vi "Que Notifier send.vi"() -> ()   [LabVIEW 2022 SP3]
panel:
  in  "Nitification Send 2":bool
  in  "error in (no error)":errorcluster
  in  "stop":bool
  out "error out":errorcluster
  out "Sent Que":i32[](array[numeric])
  out "Sent Notifier":u8
  in  "Que Send":bool
  in  "Nitification Send":bool
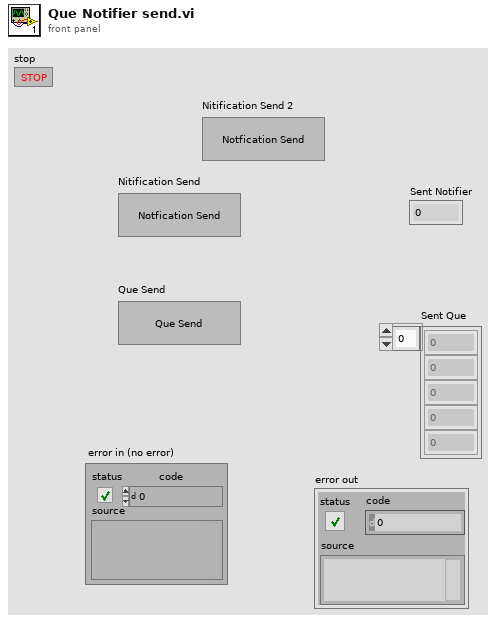
[diagram p1: front panel]
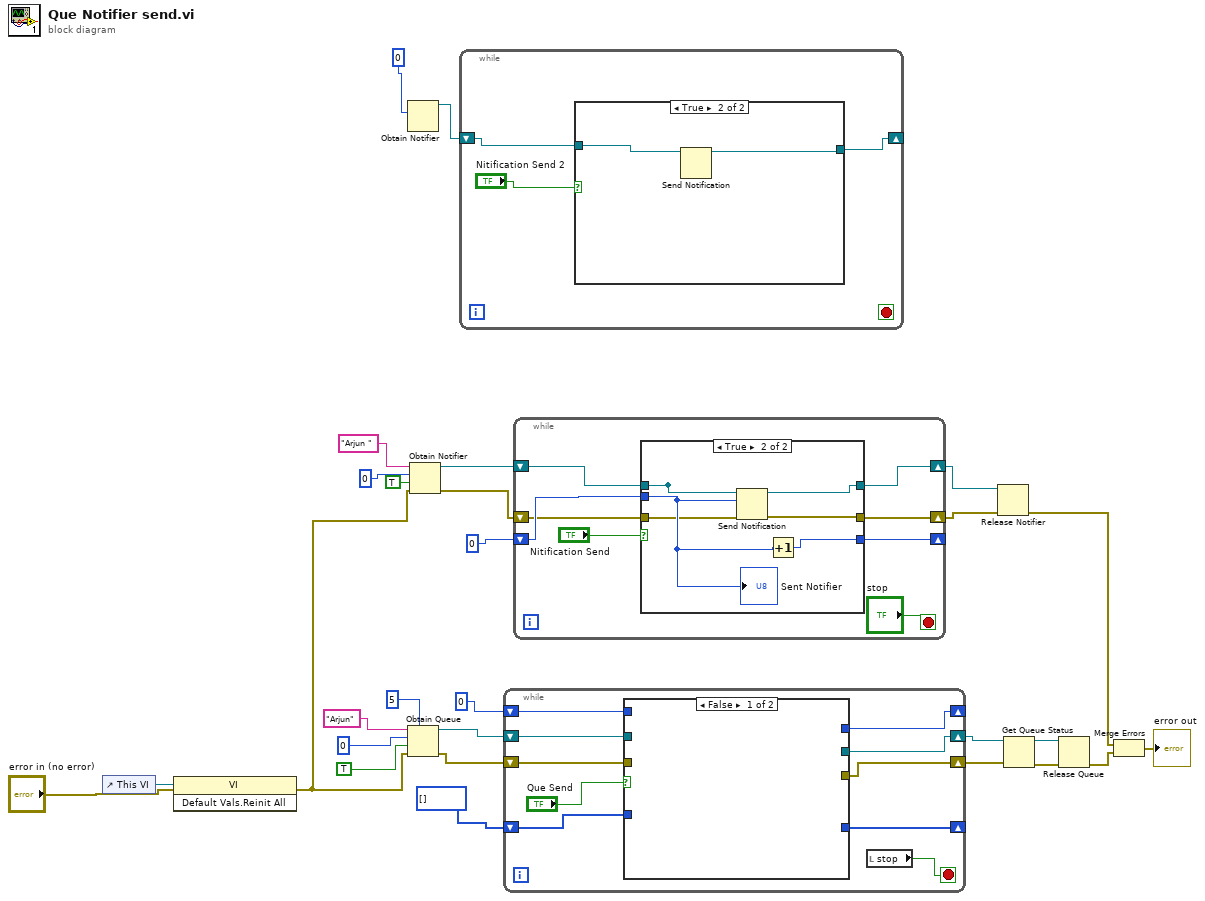
[diagram p0: block diagram]
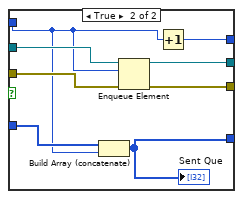
[diagram p3: hidden frame]
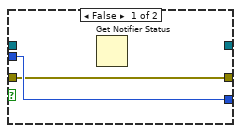
[diagram p4: hidden frame]
diagram:
  n1 = control-ref of="This VI"() -> (w10:refnum<vi>)
  n2 = invoke class="VI" method="Default Vals.Reinit All"(reference=w10, error in="error in (no error)") -> (error out=w9:errorcluster)  [unwired: 1 in, 2 out]
  n3 = Obtain Notifier(notification data type=0) -> (notifier out=w1:refnum<notifier>)  [unwired: 3 in, 2 out]
  n4 = Obtain Queue(max queue size (-1, unlimited)=5, name (unnamed)="Arjun", element data type=0, create if not found? (T)=TRUE, error in (no error)=w9) -> (queue out=w25:refnum<queue>, error out=w24:errorcluster)  [unwired: 1 out]
  n5 = Obtain Notifier(name (unnamed)="Arjun ", notification data type=0, create if not found? (T)=TRUE, error in (no error)=w9) -> (notifier out=w3:refnum<notifier>, error out=w8:errorcluster)  [unwired: 1 out]
  n6 = while {
    shift-right: [w29] -> _
    shift-left: w1 -> [w30]
    stop <- _ stop-if-true
    n7 = case shown="True" "Nitification Send 2" {
      tunnel: w30 -> [w32 w34]
      tunnel: [w32 w33] -> _
      tunnel: [w32 _] -> w29
      frame False {
      }
      frame True {
        n8 = Send Notification(notifier=w34) -> (notifier out=w33:refnum<notifier>)  [unwired: 2 in, 1 out]
      }
    }
  }
  n9 = while {
    shift-right: [w41] -> w18
    shift-left: w25 -> [w43]
    shift-right: [w40] -> w17
    shift-left: w24 -> [w42]
    shift-right: [w36] -> _
    shift-left: i32[] [] -> [w39]
    shift-right: [w37] -> _
    shift-left: 0 -> [w38]
    stop <- w35 stop-if-true
    n10 = case shown="False" "Que Send" {
      tunnel: w43 -> [_ w52]
      tunnel: w42 -> [_ w51]
      tunnel: [_ w50] -> w41
      tunnel: [_ w49] -> w40
      tunnel: w39 -> [_ w48]
      tunnel: w38 -> [_ w47]
      tunnel: [_ w46] -> w37
      tunnel: [_ w45] -> w36
      frame False {
      }
      frame True {
        n11 = Build Array (concatenate)(w48, w47) -> (w45:i32[])
        "Sent Que" <- w45
        n12 = Enqueue Element(queue=w52, element=w47, error in (no error)=w51) -> (queue out=w50:refnum<queue>, error out=w49:errorcluster)  [unwired: 1 in, 1 out]
        n13 = Increment(x=w47) -> (x+1=w46:i32)
      }
    }
    n14 = local read "stop"() -> (w35:bool)
  }
  n15 = while {
    shift-right: [w57] -> w26
    shift-left: w3 -> [w60]
    shift-right: [w56] -> _
    shift-left: 0 -> [w58]
    shift-right: [w53] -> w7
    shift-left: w8 -> [w54]
    stop <- "stop" stop-if-true
    n16 = case shown="True" "Nitification Send" {
      tunnel: [_ w68] -> _
      tunnel: w60 -> [_ w68]
      tunnel: w58 -> [w62 w65]
      tunnel: [_ w67] -> w57
      tunnel: [w62 w66] -> w56
      tunnel: w54 -> [w61 w64]
      tunnel: [w61 w63] -> w53
      frame False {
        n17 = Get Notifier Status() -> ()  [unwired: 2 in, 5 out]
      }
      frame True {
        n18 = Send Notification(notification=w65, notifier=w68, error in (no error)=w64) -> (notifier out=w67:refnum<notifier>, error out=w63:errorcluster)
        n19 = Increment(x=w65) -> (x+1=w66:i32)
        "Sent Notifier" <- w65
      }
    }
  }
  n20 = Release Notifier(notifier=w26, error in (no error)=w7) -> (error out=w13:errorcluster)  [unwired: 1 in, 2 out]
  n21 = Get Queue Status(queue=w18, error in (no error)=w17) -> (queue out=w16:refnum<queue>, error out=w15:errorcluster)  [unwired: 1 in, 6 out]
  n22 = Release Queue(queue=w16, error in (no error)=w15) -> (error out=w14:errorcluster)  [unwired: 1 in, 2 out]
  n23 = Merge Errors(w13, w14) -> (→"error out":errorcluster)
